vi "Messy Save Time Sandbox (PC).vi"() -> ()   [LabVIEW 2013]
uses:
  <vilib>/Utility/file.llb/Write To Spreadsheet File (DBL).vi
panel:
  in  "Spreadsheet Save?":bool
  out "Text Total":dbl
  out "Text":dbl[](array[numeric])
  out "Sheet":dbl[](array[numeric])
  out "Sheet Total":dbl
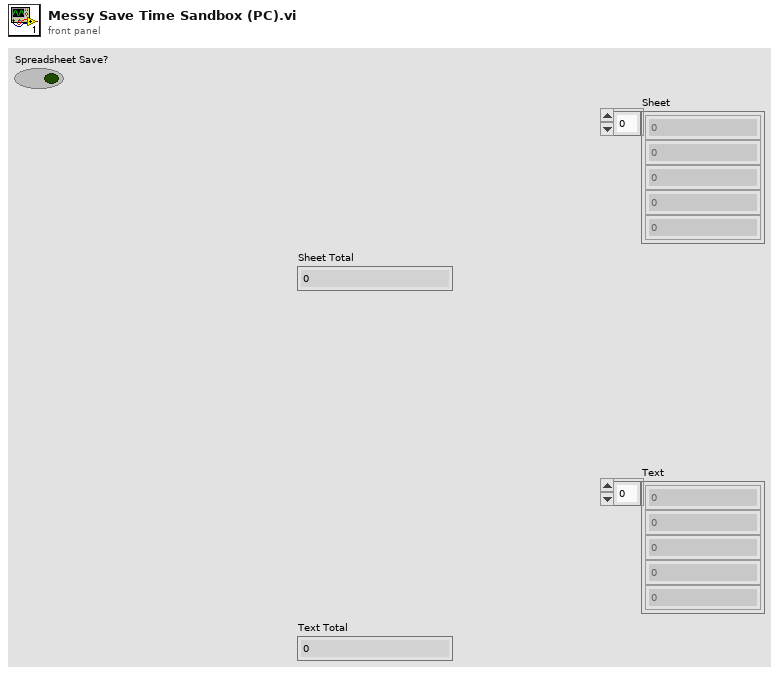
[diagram p1: front panel]
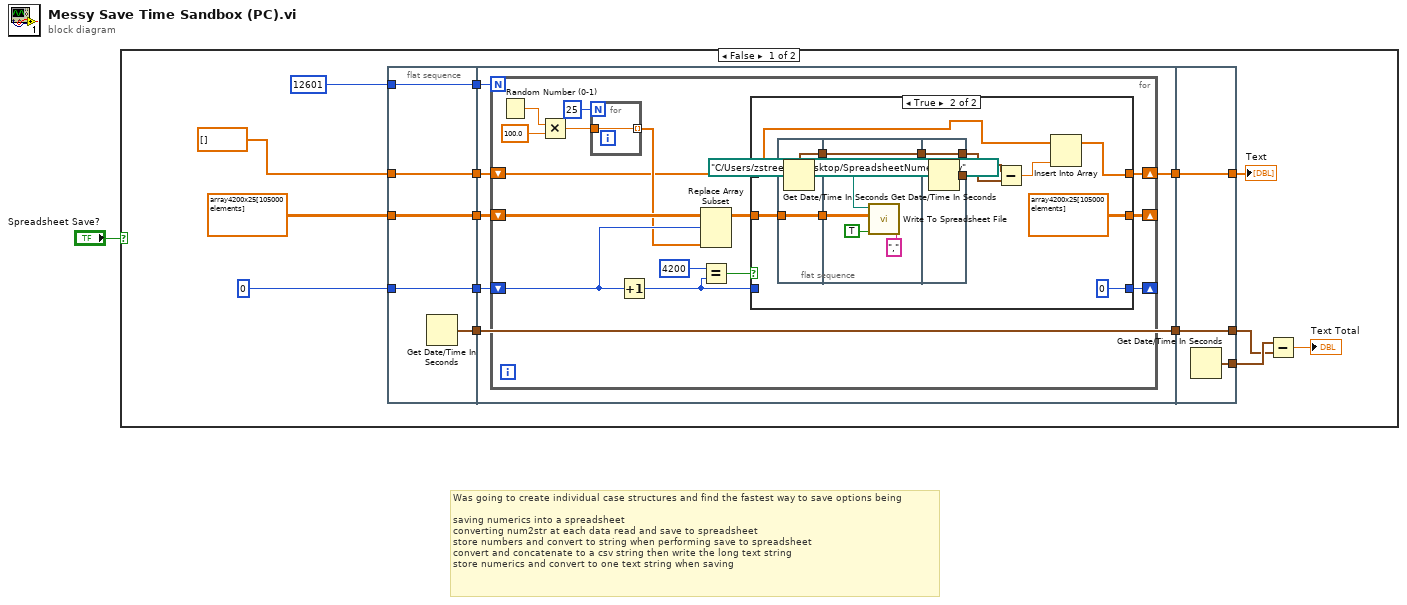
[diagram p0: block diagram]
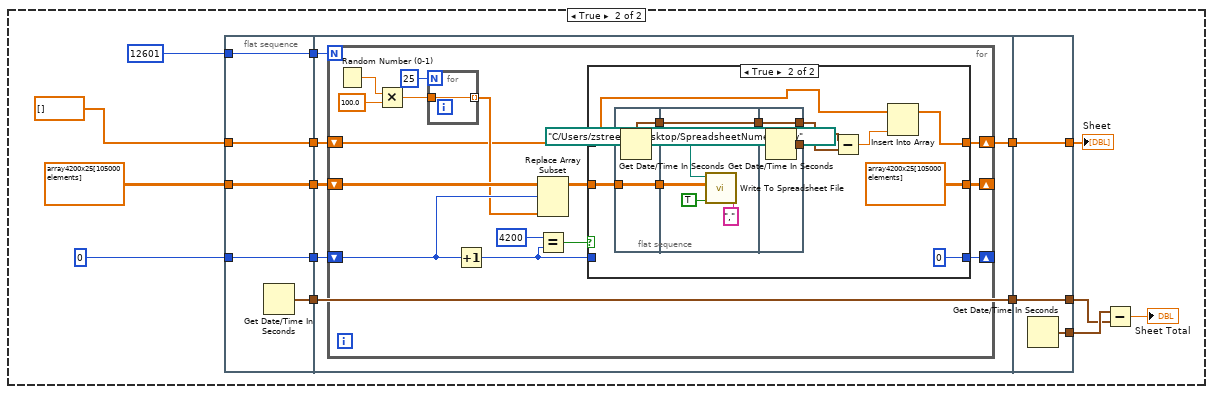
[diagram p3: hidden frame]
diagram:
  # "Was going to create individual case structures and find the fastest way to save options being\n\nsaving numerics into a spreadsheet\nconverting num2str at each data read and save to spreadsheet\nstore numbers and convert to string when performing save to spreadsheet\nconvert and concatenate to a csv string then write the long text string\nstore numerics and convert to one text string when saving"
  n1 = case shown="False" "Spreadsheet Save?" {
    frame False {
      n2 = flat-sequence {
        tunnel: dbl[] [] -> [w18]
        tunnel: 0 -> [w19]
        tunnel: dbl[][] array4200x25[105000 elements] -> [w20]
        tunnel: 12601 -> [w21]
        tunnel: [w21] -> w16
        tunnel: [w20] -> w15
        tunnel: [w19] -> w14
        tunnel: [w18] -> w13
        tunnel: [w17] -> w12
        tunnel: w16 -> [w27]
        tunnel: w15 -> [w26]
        tunnel: w14 -> [w25]
        tunnel: w13 -> [w24]
        tunnel: [w23] -> w11
        tunnel: w12 -> [w23]
        tunnel: [w22] -> w10
        tunnel: [w69] -> w2
        tunnel: w11 -> [w69]
        tunnel: [w68] -> w3
        tunnel: [w67] -> w4
        tunnel: w10 -> [w67]
        frame #0 {
          n3 = Get Date/Time In Seconds() -> (seconds since 1Jan1904=w17:timestamp)
        }
        frame #1 {
          n4 = for {
            N: w27 -> [_]
            shift-right: [w34] -> _
            shift-left: w26 -> [w40]
            shift-right: [w33] -> _
            shift-left: w25 -> [w39]
            shift-right: [w28] -> w22
            shift-left: w24 -> [w29]
            n5 = Random Number (0-1)() -> (number: 0 to 1=w42:dbl)
            n6 = Multiply(x=w42, y=100.0) -> (x*y=w32:dbl)
            n7 = for {
              N: 25 -> [_]
              tunnel: w32 -> [w43]
              tunnel: [w43] -> w31 mode=indexing
            }
            n8 = Increment(x=w39) -> (x+1=w36:i32)
            n9 = Replace Array Subset(array=w40, new element=w31, index (row)=w39) -> (w35:dbl[][])  [unwired: 1 in]
            n10 = Equal?(x=4200, y=w36) -> (x = y?=w37:bool)
            n11 = case shown="True" w37 {
              tunnel: w36 -> [w45 _]
              tunnel: w35 -> [w46 w55]
              tunnel: [w46 dbl[][] array4200x25[105000 elements]] -> w34
              tunnel: [w45 0] -> w33
              tunnel: [w44 w50] -> w28
              tunnel: w29 -> [w44 w51]
              frame False {
              }
              frame True {
                n12 = flat-sequence {
                  tunnel: w55 -> [w59]
                  tunnel: [w59] -> w54
                  tunnel: [w58] -> w52
                  tunnel: w54 -> [w64]
                  tunnel: [w60] -> w53
                  tunnel: w52 -> [w60]
                  tunnel: [w66] -> w48
                  tunnel: w53 -> [w66]
                  tunnel: [w65] -> w47
                  frame #0 {
                    n13 = Get Date/Time In Seconds() -> (seconds since 1Jan1904=w58:timestamp)
                  }
                  frame #1 {
                    n14 = call-poly <vilib>:"Write To Spreadsheet File.vi"("delimiter (\\t)"="," ("delimiter (\\t)"), "append to file? (new file:F)"=TRUE, "2D data"=w64, "file path (dialog if empty)"=path "C:/Users/zstreeter/Desktop/SpreadsheetNumeric.csv") -> ()  [unwired: 4 in, 1 out]
                  }
                  frame #2 {
                    n15 = Get Date/Time In Seconds() -> (seconds since 1Jan1904=w65:timestamp)
                  }
                }
                n16 = Subtract(x=w47, y=w48) -> (x-y=w49:dbl)
                n17 = Insert Into Array(array=w51, new element=w49) -> (w50:dbl[])  [unwired: 1 in]
              }
            }
          }
        }
        frame #2 {
          n18 = Get Date/Time In Seconds() -> (seconds since 1Jan1904=w68:timestamp)
        }
      }
      n19 = Subtract(x=w3, y=w2) -> (x-y=→"Text Total":dbl)
      "Text" <- w4
    }
    frame True {
      n20 = flat-sequence {
        tunnel: dbl[] [] -> [w86]
        tunnel: 0 -> [w87]
        tunnel: dbl[][] array4200x25[105000 elements] -> [w88]
        tunnel: 12601 -> [w89]
        tunnel: [w89] -> w84
        tunnel: [w88] -> w83
        tunnel: [w87] -> w82
        tunnel: [w86] -> w81
        tunnel: [w85] -> w80
        tunnel: w84 -> [w95]
        tunnel: w83 -> [w94]
        tunnel: w82 -> [w93]
        tunnel: w81 -> [w92]
        tunnel: [w91] -> w79
        tunnel: w80 -> [w91]
        tunnel: [w90] -> w78
        tunnel: [w137] -> w70
        tunnel: w79 -> [w137]
        tunnel: [w136] -> w71
        tunnel: [w135] -> w72
        tunnel: w78 -> [w135]
        frame #0 {
          n21 = Get Date/Time In Seconds() -> (seconds since 1Jan1904=w85:timestamp)
        }
        frame #1 {
          n22 = for {
            N: w95 -> [_]
            shift-right: [w102] -> _
            shift-left: w94 -> [w108]
            shift-right: [w101] -> _
            shift-left: w93 -> [w107]
            shift-right: [w96] -> w90
            shift-left: w92 -> [w97]
            n23 = Random Number (0-1)() -> (number: 0 to 1=w110:dbl)
            n24 = Multiply(x=w110, y=100.0) -> (x*y=w100:dbl)
            n25 = for {
              N: 25 -> [_]
              tunnel: w100 -> [w111]
              tunnel: [w111] -> w99 mode=indexing
            }
            n26 = Increment(x=w107) -> (x+1=w104:i32)
            n27 = Replace Array Subset(array=w108, new element=w99, index (row)=w107) -> (w103:dbl[][])  [unwired: 1 in]
            n28 = Equal?(x=4200, y=w104) -> (x = y?=w105:bool)
            n29 = case shown="True" w105 {
              tunnel: w104 -> [w113 _]
              tunnel: w103 -> [w114 w123]
              tunnel: [w114 dbl[][] array4200x25[105000 elements]] -> w102
              tunnel: [w113 0] -> w101
              tunnel: [w112 w118] -> w96
              tunnel: w97 -> [w112 w119]
              frame False {
              }
              frame True {
                n30 = flat-sequence {
                  tunnel: w123 -> [w127]
                  tunnel: [w127] -> w122
                  tunnel: [w126] -> w120
                  tunnel: w122 -> [w132]
                  tunnel: [w128] -> w121
                  tunnel: w120 -> [w128]
                  tunnel: [w134] -> w116
                  tunnel: w121 -> [w134]
                  tunnel: [w133] -> w115
                  frame #0 {
                    n31 = Get Date/Time In Seconds() -> (seconds since 1Jan1904=w126:timestamp)
                  }
                  frame #1 {
                    n32 = call-poly <vilib>:"Write To Spreadsheet File.vi"("delimiter (\\t)"="," ("delimiter (\\t)"), "append to file? (new file:F)"=TRUE, "2D data"=w132, "file path (dialog if empty)"=path "C:/Users/zstreeter/Desktop/SpreadsheetNumeric.csv") -> ()  [unwired: 4 in, 1 out]
                  }
                  frame #2 {
                    n33 = Get Date/Time In Seconds() -> (seconds since 1Jan1904=w133:timestamp)
                  }
                }
                n34 = Subtract(x=w115, y=w116) -> (x-y=w117:dbl)
                n35 = Insert Into Array(array=w119, new element=w117) -> (w118:dbl[])  [unwired: 1 in]
              }
            }
          }
        }
        frame #2 {
          n36 = Get Date/Time In Seconds() -> (seconds since 1Jan1904=w136:timestamp)
        }
      }
      n37 = Subtract(x=w71, y=w70) -> (x-y=→"Sheet Total":dbl)
      "Sheet" <- w72
    }
  }
